vi "GEA2MessageFormatter.vi"(0 "Prefix(Send/Recv)":string, 7 "GEA2 Data In":T1 {"Command" format="%02x"; "Destination" format="%02x"; "Source" format="%02x"}, 11 "Error In":errorcluster) -> (4 "Output String":string, 15 "Error Out":errorcluster)   [LabVIEW 2016, in "GEA2_Toolkit.lvlib"]
uses:
  library/GEA2_Toolkit.lvlib
  type defs/Data In.ctl
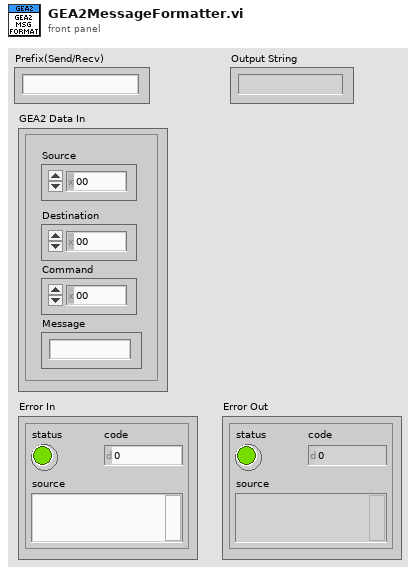
[diagram p1: front panel]
types:
  T1 = typedef "GEA2_Toolkit.lvlib/Data In.ctl" = cluster{"Source":u8, "Destination":u8, "Command":u8, "Message":string}
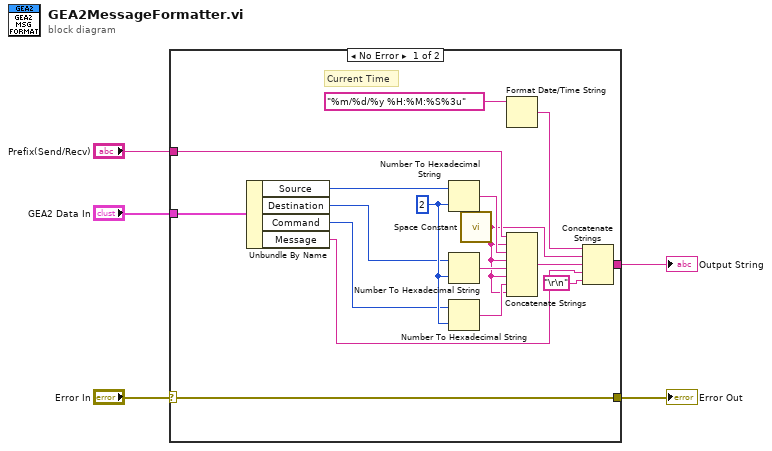
[diagram p0: block diagram]
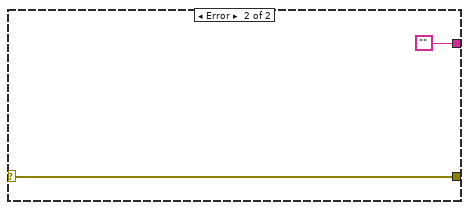
[diagram p2: hidden frame]
diagram:
  n1 = case shown="No Error" "Error In" {
    selector: "Error In" -> [w7 w24]
    tunnel: [w19 ""] -> w5
    tunnel: "Prefix(Send/Recv)" -> [w17 _]
    tunnel: "GEA2 Data In" -> [w12 _]
    tunnel: [w7 w24] -> w1
    frame No Error {
      w18 = i16 2 ("width (-)")
      # "Current Time"
      n2 = Unbundle By Name(w12) -> ("Source"=w11:u8, "Destination"=w10:u8, "Command"=w9:u8, "Message"=w6:string)
      n3 = Number To Hexadecimal String(1:w18, 2:w11) -> (0:w14:string)
      n4 = Number To Hexadecimal String(1:w18, 2:w10) -> (0:w13:string)
      n5 = Number To Hexadecimal String(1:w18, 2:w9) -> (0:w15:string)
      n6 = call <vilib>:"Space Constant.vi"() -> ("String"=w8:string)
      n7 = Format Date/Time String(time format string (%c)="%m/%d/%y %H:%M:%S%3u") -> (date/time string=w20:string)  [unwired: 2 in]
      n8 = Concatenate Strings(w17, w8, w14, w8, w13, w8, w15, w8) -> (w16:string)
      n9 = Concatenate Strings(w20, w8, w16, w6, "\r\n") -> (w19:string)
    }
    frame Error {
    }
  }
  "Output String" <- w5
  "Error Out" <- w1
